vi "SwitchControl.vi"(8 "error in (no error)":errorcluster, 10 "file path":path=path "D:/Minecraft/mmc-stable-win32/MultiMC/instances/TRAINS 4/.minecraft/saves/IR Jernbane 29.03.20/opencomputers/3ab9ee3d-68ca-49df-a255-ef05ac85667b/home") -> (0 "error out":errorcluster)   [LabVIEW 2014]
uses:
  Libraries/Map Data Folder/Map Data.lvlib
  Libraries/Contact Data/Contact Data.lvlib
panel:
  in  "Switch Find Range":dbl=15.0
  out "file path 2":path=path "D:/Minecraft/mmc-stable-win32/MultiMC/instances/TRAINS 3-/.minecraft/saves/trains/opencomputers/62f872ae-9a17-46b3-a447-fd98d4ae8740/home"
  out "file path 4":path=path "D:/Minecraft/mmc-stable-win32/MultiMC/instances/TRAINS 4/.minecraft/saves/IR Jernbane 29.03.20/opencomputers/8af95667-0df0-47dc-89ed-42af1a81d2d5/home"
  in  "Switch to Train Range":dbl=100.0
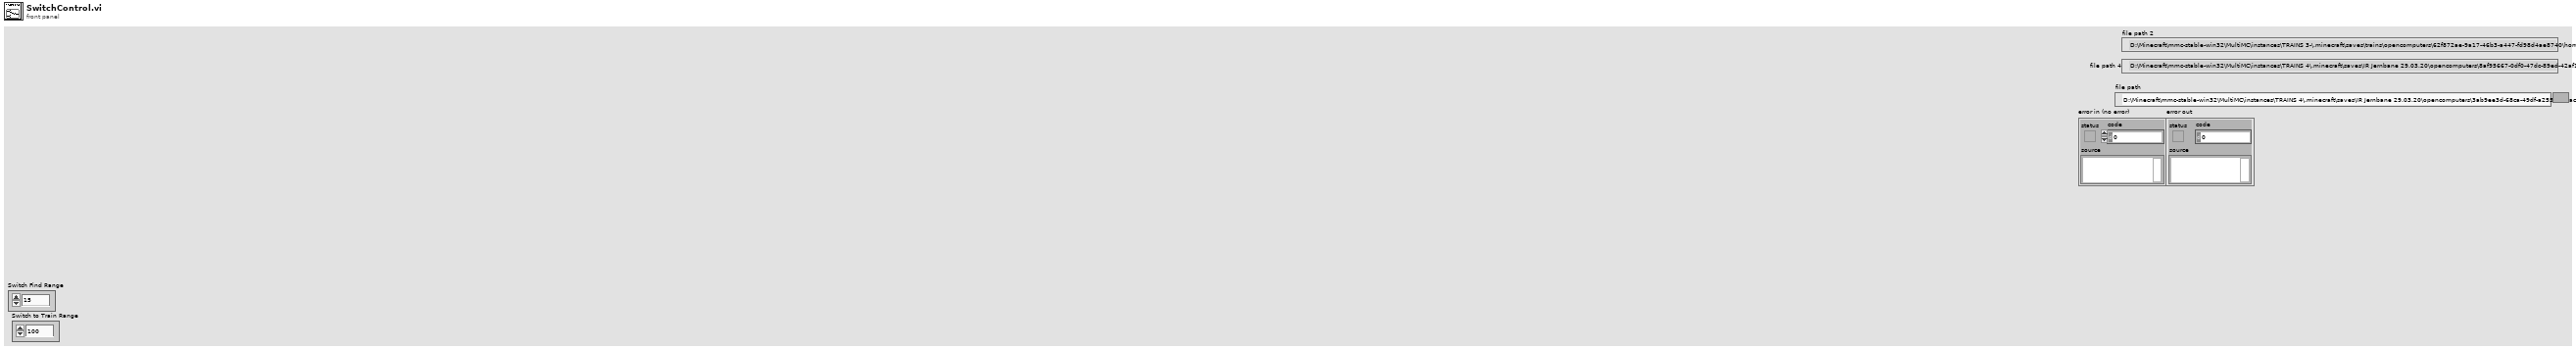
[diagram p1: front panel]
types:
  T1 = typedef "Map Data.lvlib/All-Lines.ctl" = T2[]
  T2 = typedef "Map Data.lvlib/LineCluster.ctl" = cluster{"Line name":string, "Line array":cluster{"X":dbl, "Y":dbl, "Z":dbl}[], "Line connections":T3[]}
  T3 = typedef "Map Data.lvlib/LineConnection.ctl" = cluster{"Index":i32, "Switch Pos":cluster{"X":dbl, "Y":dbl, "Z":dbl}, "Switch operational":bool, "Switch State":bool, "Connection Index":i32, "Connection Pos":cluster{"X":dbl, "Y":dbl, "Z":dbl}, "LinePos Index":i32, "ConnectPos Index":i32, "Same direction?":bool, "Manual Overide":bool, "Manual State":bool}
  T4 = typedef "Contact Data.lvlib/Contact.ctl" = cluster{"ID":u32, "UUID":string, "Name":string, "Iteration":i32, "Posit Array":T5[], "Controls":T6, "DestArray":T7[], "SetSpeed":dbl, "Speed":dbl, "PathData":T9}
  T5 = typedef "Contact Data.lvlib/Position.ctl" = cluster{"X":dbl, "Y":dbl, "Z":dbl}
  T6 = typedef "Contact Data.lvlib/Controls.ctl" = cluster{"throttle":dbl, "brake":dbl, "horn":dbl, "wait":dbl}
  T7 = typedef "Contact Data.lvlib/DestinationCluster.ctl" = cluster{"Desination":string, "DestControls":T8, "Timer":u32, "Set Timer":u32, "Time Stamp":timestamp, "Repeat?":bool, "Optional Data":string, "Distance":dbl}
  T8 = typedef "Contact Data.lvlib/DesinationControls.ctl" = enum16{"Tracker", "Manual", "Stop", "Station DateTime", "Station Timer", "Maintain"}
  T9 = typedef "Contact Data.lvlib/PathData.ctl" = cluster{"Path Found?":bool, "Same Line +Dir?":bool, "Path":T10[]}
  T10 = typedef "PathControl.ctl" = cluster{"Line Index":i32, "Line Pos Index ":i32, "Prev Index ":i32, "Prev Pos Index":i32}
  T11 = cluster{"Connection Index":i32, "ConnectPos Index":i32}
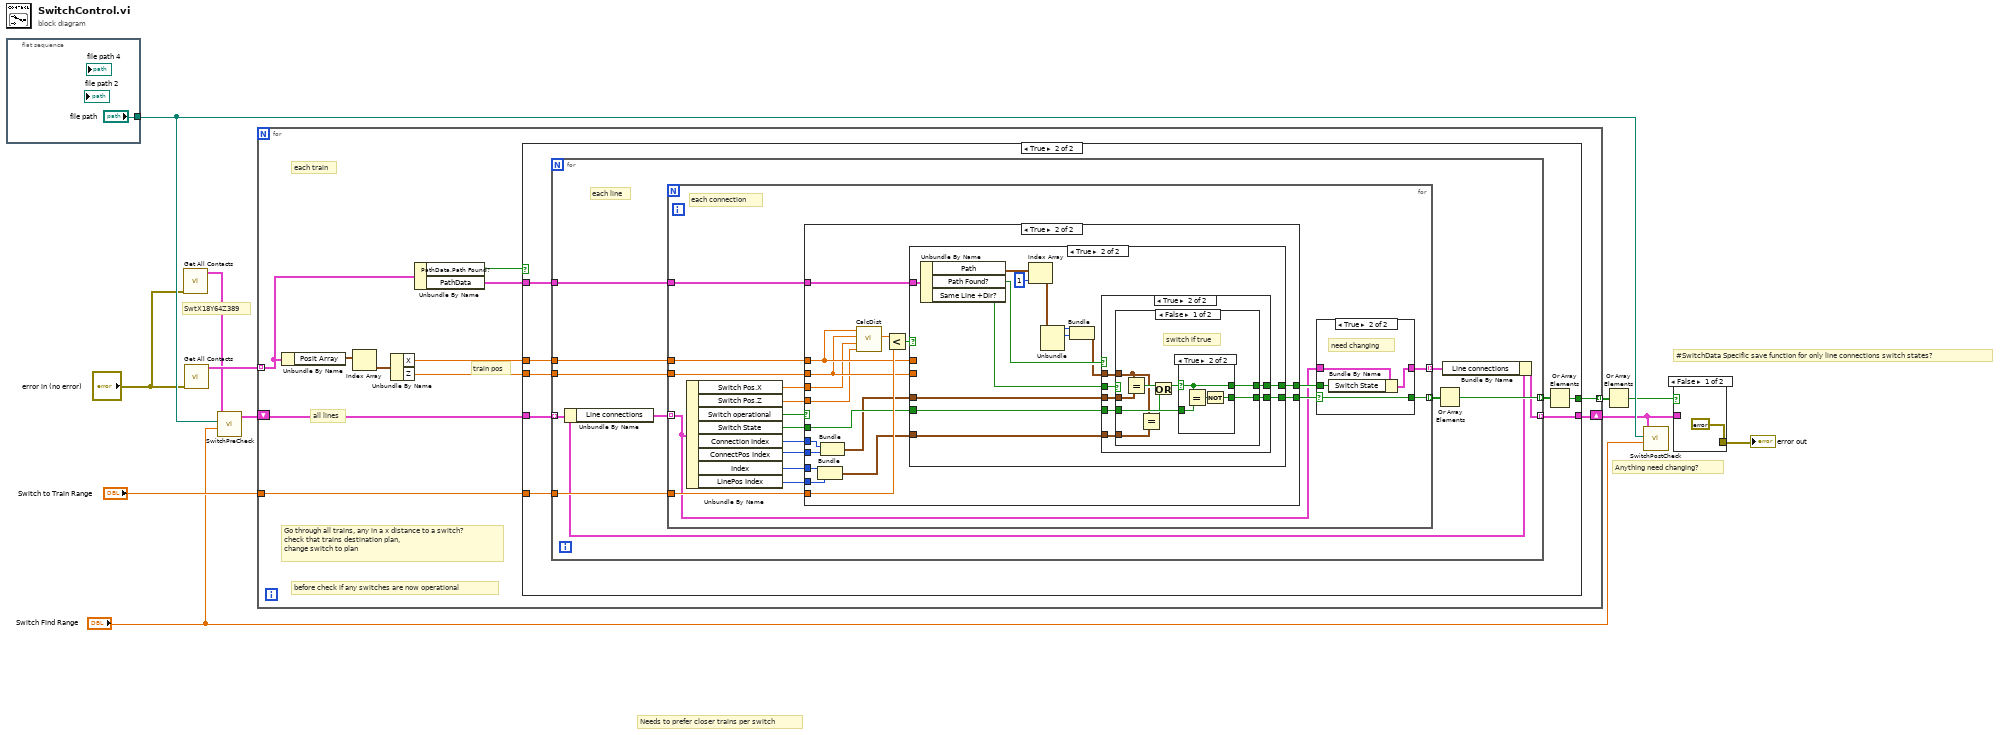
[diagram p0: block diagram]
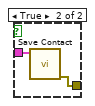
[diagram p2: hidden frame]
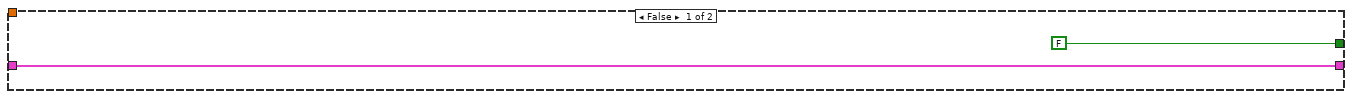
[diagram p3: hidden frame]
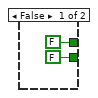
[diagram p5: hidden frame]
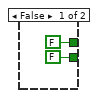
[diagram p6: hidden frame]
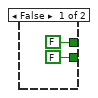
[diagram p7: hidden frame]
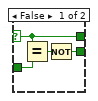
[diagram p8: hidden frame]
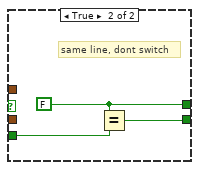
[diagram p9: hidden frame]
diagram:
  # "#SwitchData Specific save function for only line connections switch states?"
  # "Anything need changing?"
  # "SwtX18Y64Z389"
  # "Needs to prefer closer trains per switch"
  n1 = flat-sequence {
    tunnel: ["file path"] -> w11
    frame #0 {
    }
  }
  n2 = call "Get All Contacts.vi"("error in (no error)"="error in (no error)") -> ("All Lines out"=w7:T1)  [unwired: 8 in, 2 out]
  n3 = call "Get All Contacts.vi"("error in (no error)"="error in (no error)") -> ("Contacts"=w8:T4[])  [unwired: 9 in, 1 out]
  n4 = call "SwitchPreCheck.vi"("Max Dist"="Switch Find Range", "file path"=w11, "All Lines in"=w7) -> ("All Lines out"=w5:T1)  [unwired: 8 in]
  n5 = for {
    tunnel: w8 -> [w17] mode=indexing
    shift-right: [w20] -> w4
    shift-left: w5 -> [w21]
    tunnel: [w19] -> w6 mode=indexing
    tunnel: "Switch to Train Range" -> [w18]
    # "before check if any switches are now operational"
    # "train pos"
    # "Go through all trains, any in a x distance to a switch?\ncheck that trains destination plan,\nchange switch to plan"
    # "all lines"
    # "each train"
    n6 = Unbundle By Name(w17) -> ("Posit Array"=w15:T5[])
    n7 = Index Array(array=w15) -> (element=w16:T5)  [unwired: 1 in]
    n8 = Unbundle By Name(w16) -> ("X"=w23:dbl, "Z"=w22:dbl)
    n9 = Unbundle By Name(w17) -> ("PathData.Path Found?"=w14:bool, "PathData"=w13:T9)
    n10 = case shown="True" w14 {
      tunnel: w23 -> [_ w33]
      tunnel: w22 -> [_ w32]
      tunnel: w18 -> [_ w31]
      tunnel: w21 -> [w25 w30]
      tunnel: [w25 w28] -> w20
      tunnel: [FALSE w27] -> w19
      tunnel: w13 -> [_ w26]
      frame False {
      }
      frame True {
        n11 = for {
          tunnel: w30 -> [w36] mode=indexing
          tunnel: w33 -> [w42]
          tunnel: w32 -> [w41]
          tunnel: w31 -> [w40]
          tunnel: [w35] -> w28 mode=indexing
          tunnel: [w38] -> w29 mode=indexing
          tunnel: w26 -> [w34]
          # "each line"
          n12 = Unbundle By Name(w36) -> ("Line connections"=w43:T3[])
          n13 = for {
            tunnel: w43 -> [w50] mode=indexing
            tunnel: w42 -> [w60]
            tunnel: w41 -> [w59]
            tunnel: w40 -> [w55]
            tunnel: [w49] -> w37 mode=indexing
            tunnel: [w48] -> w39 mode=indexing
            tunnel: w34 -> [w44]
            # "each connection"
            n14 = Unbundle By Name(w50) -> ("Switch Pos.X"=w58:dbl, "Switch Pos.Z"=w57:dbl, "Switch operational"=w56:bool, "Switch State"=w54:bool, "Connection Index"=w53:i32, "ConnectPos Index"=w47:i32, "Index"=w46:i32, "LinePos Index"=w45:i32)
            n15 = case shown="True" w56 {
              tunnel: w60 -> [_ w82]
              tunnel: w59 -> [_ w81]
              tunnel: w58 -> [_ w80]
              tunnel: w57 -> [_ w79]
              tunnel: w55 -> [_ w84]
              tunnel: w54 -> [_ w78]
              tunnel: w53 -> [_ w74]
              tunnel: [FALSE w77] -> w52
              tunnel: [FALSE ("x") w76] -> w51
              tunnel: w47 -> [_ w75]
              tunnel: w46 -> [_ w72]
              tunnel: w45 -> [_ w71]
              tunnel: w44 -> [_ w69]
              frame False {
              }
              frame True {
                n16 = Bundle("Index"=w72, "LinePos Index"=w71) -> (w70:cluster{"Index":i32, "LinePos Index":i32})  [unwired: 1 in]
                n17 = Bundle("Connection Index"=w74, "ConnectPos Index"=w75) -> (w73:T11)  [unwired: 1 in]
                n18 = call "CalcDist.vi"("Y2"=w79, "X2"=w80, "Y1"=w81, "X1"=w82) -> ("Distance"=w85:dbl)  [unwired: 7 in]
                n19 = Less?(x=w85, y=w84) -> (x < y?=w83:bool)
                n20 = case shown="True" w83 {
                  tunnel: w82 -> [_ _]
                  tunnel: w81 -> [_ _]
                  tunnel: w73 -> [_ w101]
                  tunnel: w78 -> [_ w100]
                  tunnel: [FALSE w99] -> w77
                  tunnel: [FALSE ("x") w98] -> w76
                  tunnel: w70 -> [_ w97]
                  tunnel: w69 -> [_ w96]
                  frame False {
                  }
                  frame True {
                    n21 = Unbundle By Name(w96) -> ("Path"=w95:T10[], "Path Found?"=w92:bool, "Same Line +Dir?"=w93:bool)
                    n22 = Index Array(array=w95, index=1) -> (element=w91:T10)
                    n23 = Unbundle(w91) -> ("Line Index"=w90:i32, "Line Pos Index"=w89:i32)  [unwired: 2 out]
                    n24 = Bundle("Line Index"=w90, "Line Pos Index"=w89) -> (w88:cluster{"Line Index":i32, "Line Pos Index ":i32})  [unwired: 1 in]
                    n25 = case shown="True" w92 {
                      tunnel: w88 -> [_ w110]
                      tunnel: w101 -> [_ w109]
                      tunnel: w93 -> [_ w108]
                      tunnel: w100 -> [_ w107]
                      tunnel: [FALSE w106] -> w99
                      tunnel: [FALSE ("x") w105] -> w98
                      tunnel: w97 -> [_ w104]
                      frame False {
                      }
                      frame True {
                        n26 = case shown="False" w108 {
                          tunnel: w110 -> [w114 _]
                          tunnel: w109 -> [w119 _]
                          tunnel: w107 -> [w118 w130]
                          tunnel: [w117 w128] -> w106
                          tunnel: [w116 w129] -> w105
                          tunnel: w104 -> [w113 _]
                          frame False {
                            # "switch if true"
                            n27 = Equal?(x=w114, y=w119) -> (x = y?=w115:bool)
                            n28 = Equal?(x=w114, y=w113) -> (x = y?=w111:bool)
                            n29 = Or(x=w115, y=w111) -> (x .or. y?=w112:bool)
                            n30 = case shown="True" w112 {
                              selector: w112 -> [w121 w125]
                              tunnel: w118 -> [w123 w127]
                              tunnel: [w120 w124] -> w117
                              tunnel: [w121 w125] -> w116
                              frame False {
                                n31 = Equal?(x=w121, y=w123) -> (x = y?=w122:bool)
                                n32 = Not(x=w122) -> (.not. x?=w120:bool)
                              }
                              frame True {
                                n33 = Equal?(x=w125, y=w127) -> (x = y?=w126:bool)
                                n34 = Not(x=w126) -> (.not. x?=w124:bool)
                              }
                            }
                          }
                          frame True {
                            w129 = FALSE ("x")
                            # "same line, dont switch"
                            n35 = Equal?(x=w129, y=w130) -> (x = y?=w128:bool)
                          }
                        }
                      }
                    }
                  }
                }
              }
            }
            n36 = case shown="True" w52 {
              selector: w52 -> [w61 w63]
              tunnel: w51 -> [_ w66]
              tunnel: w50 -> [w62 w65]
              tunnel: [w62 w64] -> w49
              tunnel: [w61 w63] -> w48
              frame False {
              }
              frame True {
                # "need changing"
                n37 = Bundle By Name(cluster=w65, "Switch State"=w66) -> (w64:T3)
              }
            }
          }
          n38 = Or Array Elements(Boolean array=w39) -> (logical OR=w38:bool)
          n39 = Bundle By Name(cluster=w36, "Line connections"=w37) -> (w35:T2)
        }
        n40 = Or Array Elements(Boolean array=w29) -> (logical OR=w27:bool)
      }
    }
  }
  n41 = Or Array Elements(Boolean array=w6) -> (logical OR=w3:bool)
  n42 = call "SwitchPostCheck.vi"("Max Distance"="Switch Find Range", "file path"=w11, "All Lines in"=w4) -> ()  [unwired: 9 in]
  n43 = case shown="False" w3 {
    tunnel: w4 -> [_ w133]
    tunnel: [errorcluster {"status"=FALSE, "code"=0, "source"=""} ("error out") w132] -> w1
    frame False {
    }
    frame True {
      n44 = call "Save Contact.vi"("All Lines"=w133) -> ("error out"=w132:errorcluster)  [unwired: 9 in, 1 out]
    }
  }
  "error out" <- w1
